vi "TDT-Open Block (offline).vi"(0 "Data":T1={"TTankX"=refnum, "TDevAccX"=refnum, "LastTime"=0.0, "error"={"status"=FALSE, "code"=0, "source"=""}, "Block Name"="", "Circuit Tag"="", "Tank Name"="", "NumTicks"=0, "LastTick"=0.0, "Idle?"=FALSE, "Wait (ms)"=1000, "LastArtf"=0.0, "LastTosc"=0.0}, 5 "Tank Name":string, 7 "Block Name":string, 11 "error in (no error)":errorcluster) -> (4 "Data (out)":T1={"TTankX"=refnum, "TDevAccX"=refnum, "LastTime"=0.0, "error"={"status"=FALSE, "code"=0, "source"=""}, "Block Name"="", "Circuit Tag"="", "Tank Name"="", "NumTicks"=0, "LastTick"=0.0, "Idle?"=FALSE, "Wait (ms)"=1000, "LastArtf"=0.0, "LastTosc"=0.0}, 15 "error out":errorcluster)   [LabVIEW 2015]
uses:
  TDT Interface Data.ctl
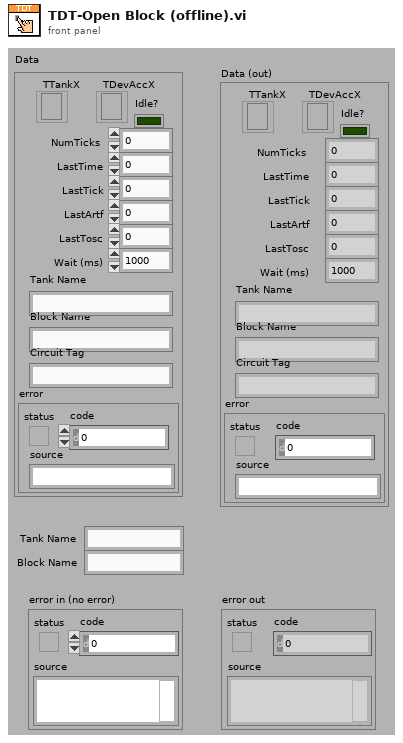
[diagram p1: front panel]
types:
  T1 = typedef "TDT Interface Data.ctl" = cluster{"TTankX":refnum<k7>, "TDevAccX":refnum<k7>, "LastTime":dbl, "error":errorcluster, "Block Name":string, "Circuit Tag":string, "Tank Name":string, "NumTicks":i32, "LastTick":dbl, "Idle?":bool, "Wait (ms)":u32, "LastArtf":dbl, "LastTosc":dbl}
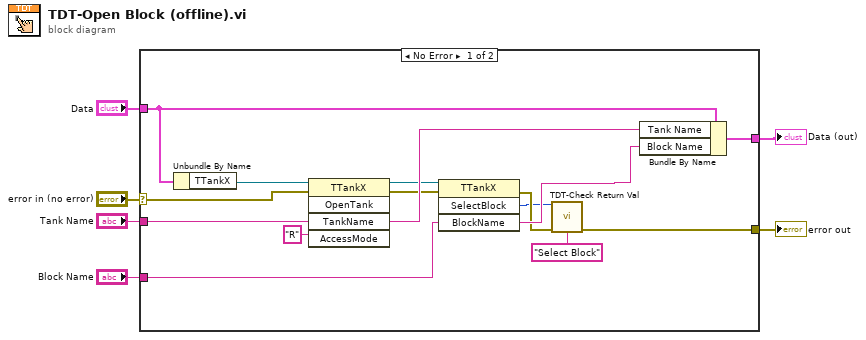
[diagram p0: block diagram]
diagram:
  n1 = case shown="No Error" "error in (no error)" {
    selector: "error in (no error)" -> [w20 w23]
    tunnel: [w21 w23] -> w5
    tunnel: "Data" -> [w18 w22]
    tunnel: [w17 w22] -> w3
    tunnel: "Tank Name" -> [w13 _]
    tunnel: "Block Name" -> [w7 _]
    frame No Error {
      n2 = Unbundle By Name(w18) -> ("TTankX"=w19:refnum<k7>)
      n3 = invoke class="TTankX" method="OpenTank"(reference=w19, error in=w20, "TankName"=w13, "AccessMode"="R") -> (reference out=w9:refnum<k7>, error out=w8:errorcluster, "TankName"=w15:string)  [unwired: 1 in, 2 out]
      n4 = invoke class="TTankX" method="SelectBlock"(reference=w9, error in=w8, "BlockName"=w7) -> (error out=w11:errorcluster, "SelectBlock"=w10:i32, "BlockName"=w14:string)  [unwired: 1 in, 1 out]
      n5 = call "TDT-Check Return Val.vi"("Return Val"=w10, "error in (no error)"=w11, "source"="Select Block" ("Message")) -> ("error out"=w21:errorcluster)  [unwired: 12 in]
      n6 = Bundle By Name(cluster=w18, "Tank Name"=w15, "Block Name"=w14) -> (w17:T1)
    }
    frame Error {
    }
  }
  "error out" <- w5
  "Data (out)" <- w3
